vi "Digitalni osciloskop.vi"() -> ()   [LabVIEW 2014]
uses:
  <instrlib>/niScope/Controls/niScope scalar measurement.ctl
  <instrlib>/niScope/Acquire/Fetch/niScope Fetch WDT.vi
panel:
  out "error out":errorcluster
  in  "error in":errorcluster
  in  "Channel":string
  out "Amplitude":dbl
  out "Min voltage":dbl
  out "Max voltage":dbl
  out "VPP":dbl
  out "Frequency":dbl
  in  "Stop Button":bool
  in  "Save plot":bool
  in  "horizontal range":dbl(knob) scale=1000.0..100000.0
  in  "vertical range":dbl(knob) scale=0.0..10.0
  in  "Filter":u16(ring) items=["Both"=3, "Lowpass filter"=1, "None"=0, "Highpass filter"=2]
  in  "Highpass filter":dbl
  in  "Lowpass filter":dbl
  in  "Freeze/Stop":bool
  out "Waveform Graph":waveform(dbl)(graph)
  in  "resource name":refnum<k15>="DAQ::1" caption="Resource name"
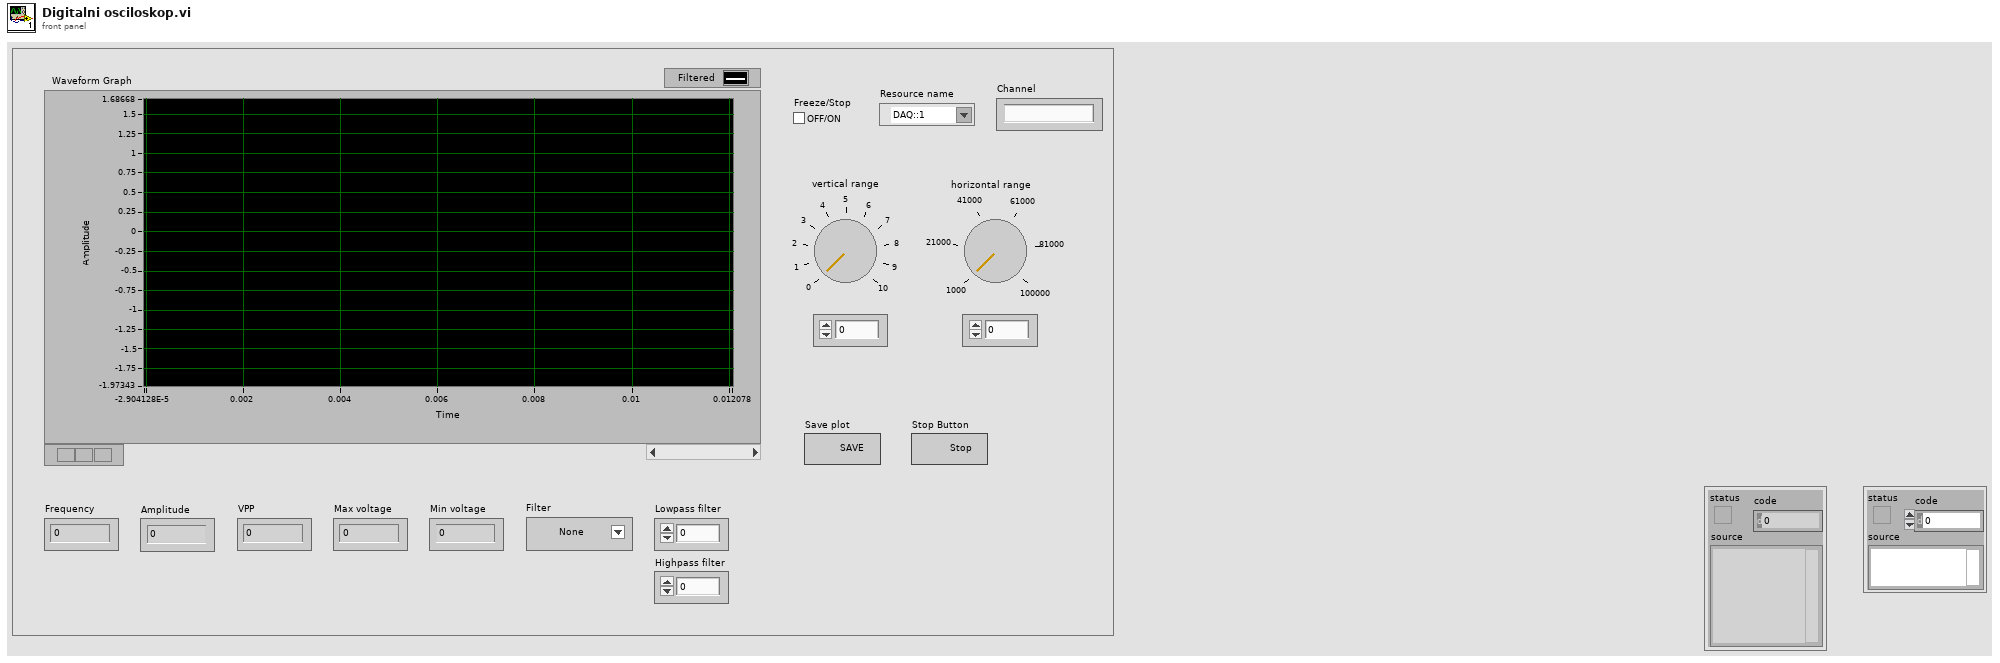
[diagram p1: front panel]
types:
  T1 = typedef "niScope scalar measurement.ctl" = i32
  T2 = typedef "imagedata.ctl" = cluster{"image type":i32, "image depth":i32, "image":u8[], "mask":u8[], "colors":u32[], "Rectangle":cluster{"left":i16, "top":i16, "right":i16, "bottom":i16}}
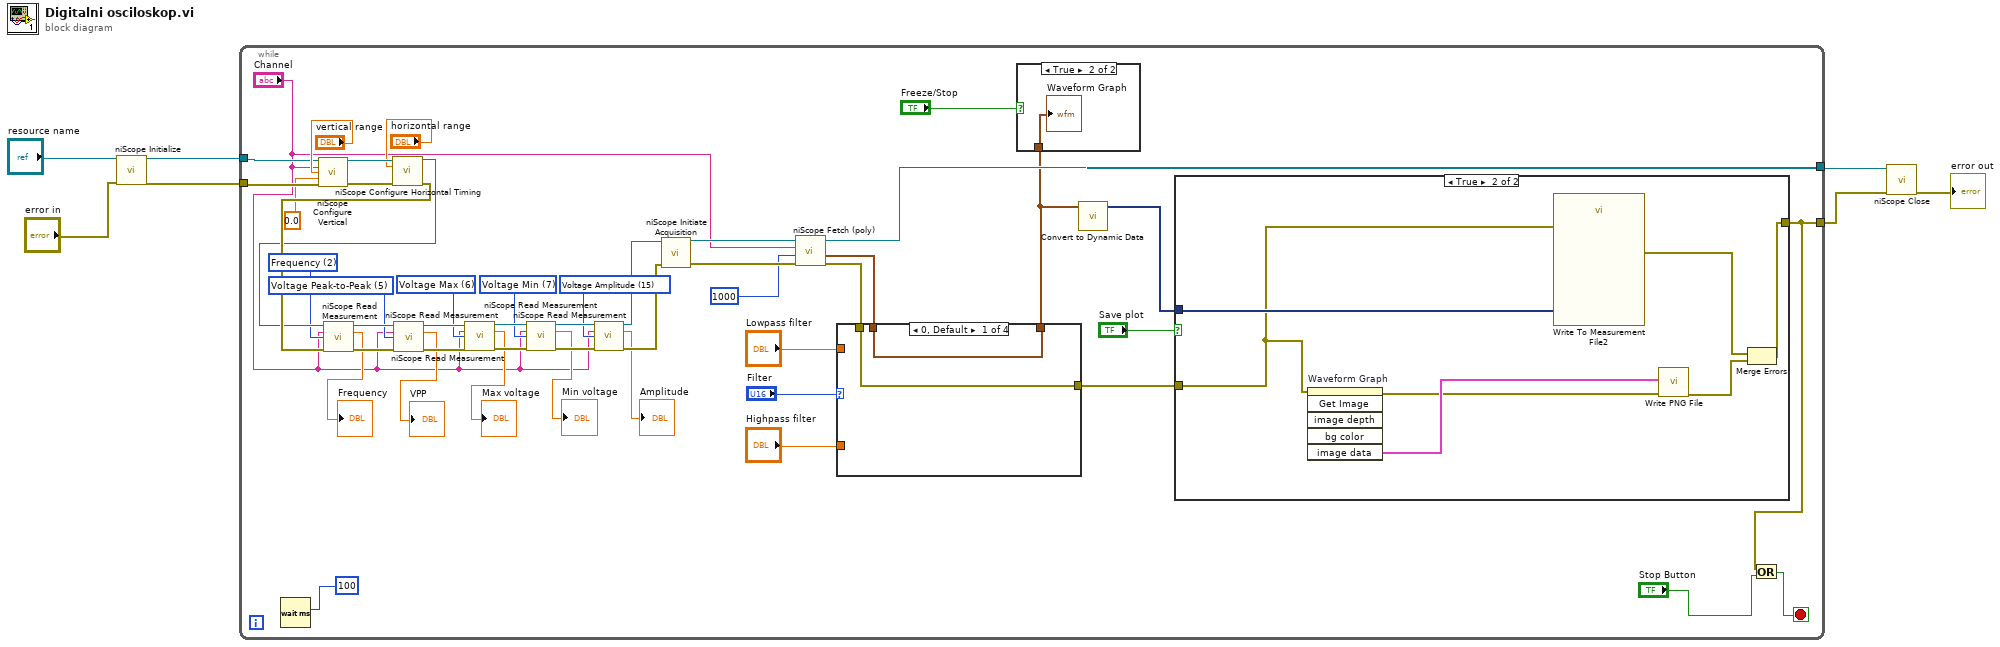
[diagram p0: block diagram]
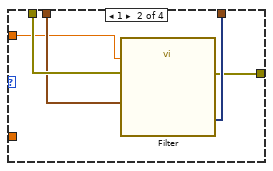
[diagram p4: hidden frame]
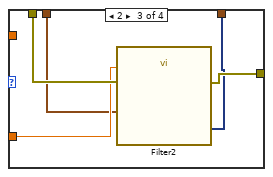
[diagram p5: hidden frame]
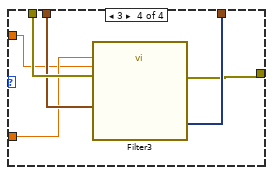
[diagram p6: hidden frame]
diagram:
  n1 = call <instrlib>:"niScope Initialize.vi"("resource name"="resource name", "error in"="error in") -> ("instrument handle"=w6:refnum<k15>, "error out"=w5:errorcluster)  [unwired: 12 in]
  n2 = while {
    tunnel: w6 -> [w43]
    tunnel: w5 -> [w44]
    tunnel: [w51] -> w4
    tunnel: [w10] -> w3
    stop <- w9 stop-if-true
    w25 = T1 15 items=["None"=4000, "Frequency"=2, "Average Frequency"=1016, "FFT Frequency"=1008, "Period"=3, "Average Period"=1015, "Rise Time"=0, "Fall Time"=1, "Rising Slew Rate"=1010, "Falling Slew Rate"=1011, "Overshoot"=18, "Preshoot"=19, "Voltage RMS"=4, "Voltage Cycle RMS"=16, "AC Estimate"=1012, "FFT Amplitude"=1009, "Voltage Average"=10, "Voltage Cycle Average"=17, "DC Estimate"=1013, "Voltage Max"=6, "Voltage Min"=7, "Voltage Peak-to-Peak"=5, "Voltage High"=8, "Voltage Low"=9, "Voltage Amplitude"=15, "Voltage Top"=1007, "Voltage Base"=1006, "Voltage Base-to-Top"=1017, "Negative Width"=11, "Positive Width"=12, "Negative Duty Cycle"=13, "Positive Duty Cycle"=14, "Integral"=1005, "Area"=1003, "Cycle Area"=1004, "Time Delay"=1014, "Phase Delay"=1018, "Low Ref Volts"=1000, "Mid Ref Volts"=1001, "High Ref Volts"=1002, "Volt. Hist. Mean"=2000, "Volt. Hist. Stdev"=2001, "Volt. Hist. Median"=2003, "Volt. Hist. Mode"=2010, "Volt. Hist. Max"=2005, "Volt. Hist. Min"=2006, "Volt. Hist. Peak-to-Peak"=2002, "Volt. Hist. Mean + Stdev"=2007, "Volt. Hist. Mean + 2 Stdev"=2008, "Volt. Hist. Mean + 3 Stdev"=2009, "Volt. Hist. Hits"=2004, "Volt. Hist. New Hits"=2011, "Time Hist. Mean"=3000, "Time Hist. Stdev"=3001, "Time Hist. Median"=3003, "Time Hist. Mode"=3010, "Time Hist. Max"=3005, "Time Hist. Min"=3006, "Time Hist. Peak-to-Peak"=3002, "Time Hist. Mean + Stdev"=3007, "Time Hist. Mean + 2 Stdev"=3008, "Time Hist. Mean + 3 Stdev"=3009, "Time Hist. Hits"=3004, "Time Hist. New Hits"=3011] ("scalar measurement")
    w26 = T1 7 items=["None"=4000, "Frequency"=2, "Average Frequency"=1016, "FFT Frequency"=1008, "Period"=3, "Average Period"=1015, "Rise Time"=0, "Fall Time"=1, "Rising Slew Rate"=1010, "Falling Slew Rate"=1011, "Overshoot"=18, "Preshoot"=19, "Voltage RMS"=4, "Voltage Cycle RMS"=16, "AC Estimate"=1012, "FFT Amplitude"=1009, "Voltage Average"=10, "Voltage Cycle Average"=17, "DC Estimate"=1013, "Voltage Max"=6, "Voltage Min"=7, "Voltage Peak-to-Peak"=5, "Voltage High"=8, "Voltage Low"=9, "Voltage Amplitude"=15, "Voltage Top"=1007, "Voltage Base"=1006, "Voltage Base-to-Top"=1017, "Negative Width"=11, "Positive Width"=12, "Negative Duty Cycle"=13, "Positive Duty Cycle"=14, "Integral"=1005, "Area"=1003, "Cycle Area"=1004, "Time Delay"=1014, "Phase Delay"=1018, "Low Ref Volts"=1000, "Mid Ref Volts"=1001, "High Ref Volts"=1002, "Volt. Hist. Mean"=2000, "Volt. Hist. Stdev"=2001, "Volt. Hist. Median"=2003, "Volt. Hist. Mode"=2010, "Volt. Hist. Max"=2005, "Volt. Hist. Min"=2006, "Volt. Hist. Peak-to-Peak"=2002, "Volt. Hist. Mean + Stdev"=2007, "Volt. Hist. Mean + 2 Stdev"=2008, "Volt. Hist. Mean + 3 Stdev"=2009, "Volt. Hist. Hits"=2004, "Volt. Hist. New Hits"=2011, "Time Hist. Mean"=3000, "Time Hist. Stdev"=3001, "Time Hist. Median"=3003, "Time Hist. Mode"=3010, "Time Hist. Max"=3005, "Time Hist. Min"=3006, "Time Hist. Peak-to-Peak"=3002, "Time Hist. Mean + Stdev"=3007, "Time Hist. Mean + 2 Stdev"=3008, "Time Hist. Mean + 3 Stdev"=3009, "Time Hist. Hits"=3004, "Time Hist. New Hits"=3011] ("scalar measurement")
    w27 = T1 6 items=["None"=4000, "Frequency"=2, "Average Frequency"=1016, "FFT Frequency"=1008, "Period"=3, "Average Period"=1015, "Rise Time"=0, "Fall Time"=1, "Rising Slew Rate"=1010, "Falling Slew Rate"=1011, "Overshoot"=18, "Preshoot"=19, "Voltage RMS"=4, "Voltage Cycle RMS"=16, "AC Estimate"=1012, "FFT Amplitude"=1009, "Voltage Average"=10, "Voltage Cycle Average"=17, "DC Estimate"=1013, "Voltage Max"=6, "Voltage Min"=7, "Voltage Peak-to-Peak"=5, "Voltage High"=8, "Voltage Low"=9, "Voltage Amplitude"=15, "Voltage Top"=1007, "Voltage Base"=1006, "Voltage Base-to-Top"=1017, "Negative Width"=11, "Positive Width"=12, "Negative Duty Cycle"=13, "Positive Duty Cycle"=14, "Integral"=1005, "Area"=1003, "Cycle Area"=1004, "Time Delay"=1014, "Phase Delay"=1018, "Low Ref Volts"=1000, "Mid Ref Volts"=1001, "High Ref Volts"=1002, "Volt. Hist. Mean"=2000, "Volt. Hist. Stdev"=2001, "Volt. Hist. Median"=2003, "Volt. Hist. Mode"=2010, "Volt. Hist. Max"=2005, "Volt. Hist. Min"=2006, "Volt. Hist. Peak-to-Peak"=2002, "Volt. Hist. Mean + Stdev"=2007, "Volt. Hist. Mean + 2 Stdev"=2008, "Volt. Hist. Mean + 3 Stdev"=2009, "Volt. Hist. Hits"=2004, "Volt. Hist. New Hits"=2011, "Time Hist. Mean"=3000, "Time Hist. Stdev"=3001, "Time Hist. Median"=3003, "Time Hist. Mode"=3010, "Time Hist. Max"=3005, "Time Hist. Min"=3006, "Time Hist. Peak-to-Peak"=3002, "Time Hist. Mean + Stdev"=3007, "Time Hist. Mean + 2 Stdev"=3008, "Time Hist. Mean + 3 Stdev"=3009, "Time Hist. Hits"=3004, "Time Hist. New Hits"=3011] ("scalar measurement")
    w28 = T1 5 items=["None"=4000, "Frequency"=2, "Average Frequency"=1016, "FFT Frequency"=1008, "Period"=3, "Average Period"=1015, "Rise Time"=0, "Fall Time"=1, "Rising Slew Rate"=1010, "Falling Slew Rate"=1011, "Overshoot"=18, "Preshoot"=19, "Voltage RMS"=4, "Voltage Cycle RMS"=16, "AC Estimate"=1012, "FFT Amplitude"=1009, "Voltage Average"=10, "Voltage Cycle Average"=17, "DC Estimate"=1013, "Voltage Max"=6, "Voltage Min"=7, "Voltage Peak-to-Peak"=5, "Voltage High"=8, "Voltage Low"=9, "Voltage Amplitude"=15, "Voltage Top"=1007, "Voltage Base"=1006, "Voltage Base-to-Top"=1017, "Negative Width"=11, "Positive Width"=12, "Negative Duty Cycle"=13, "Positive Duty Cycle"=14, "Integral"=1005, "Area"=1003, "Cycle Area"=1004, "Time Delay"=1014, "Phase Delay"=1018, "Low Ref Volts"=1000, "Mid Ref Volts"=1001, "High Ref Volts"=1002, "Volt. Hist. Mean"=2000, "Volt. Hist. Stdev"=2001, "Volt. Hist. Median"=2003, "Volt. Hist. Mode"=2010, "Volt. Hist. Max"=2005, "Volt. Hist. Min"=2006, "Volt. Hist. Peak-to-Peak"=2002, "Volt. Hist. Mean + Stdev"=2007, "Volt. Hist. Mean + 2 Stdev"=2008, "Volt. Hist. Mean + 3 Stdev"=2009, "Volt. Hist. Hits"=2004, "Volt. Hist. New Hits"=2011, "Time Hist. Mean"=3000, "Time Hist. Stdev"=3001, "Time Hist. Median"=3003, "Time Hist. Mode"=3010, "Time Hist. Max"=3005, "Time Hist. Min"=3006, "Time Hist. Peak-to-Peak"=3002, "Time Hist. Mean + Stdev"=3007, "Time Hist. Mean + 2 Stdev"=3008, "Time Hist. Mean + 3 Stdev"=3009, "Time Hist. Hits"=3004, "Time Hist. New Hits"=3011] ("scalar measurement")
    w39 = T1 2 items=["None"=4000, "Frequency"=2, "Average Frequency"=1016, "FFT Frequency"=1008, "Period"=3, "Average Period"=1015, "Rise Time"=0, "Fall Time"=1, "Rising Slew Rate"=1010, "Falling Slew Rate"=1011, "Overshoot"=18, "Preshoot"=19, "Voltage RMS"=4, "Voltage Cycle RMS"=16, "AC Estimate"=1012, "FFT Amplitude"=1009, "Voltage Average"=10, "Voltage Cycle Average"=17, "DC Estimate"=1013, "Voltage Max"=6, "Voltage Min"=7, "Voltage Peak-to-Peak"=5, "Voltage High"=8, "Voltage Low"=9, "Voltage Amplitude"=15, "Voltage Top"=1007, "Voltage Base"=1006, "Voltage Base-to-Top"=1017, "Negative Width"=11, "Positive Width"=12, "Negative Duty Cycle"=13, "Positive Duty Cycle"=14, "Integral"=1005, "Area"=1003, "Cycle Area"=1004, "Time Delay"=1014, "Phase Delay"=1018, "Low Ref Volts"=1000, "Mid Ref Volts"=1001, "High Ref Volts"=1002, "Volt. Hist. Mean"=2000, "Volt. Hist. Stdev"=2001, "Volt. Hist. Median"=2003, "Volt. Hist. Mode"=2010, "Volt. Hist. Max"=2005, "Volt. Hist. Min"=2006, "Volt. Hist. Peak-to-Peak"=2002, "Volt. Hist. Mean + Stdev"=2007, "Volt. Hist. Mean + 2 Stdev"=2008, "Volt. Hist. Mean + 3 Stdev"=2009, "Volt. Hist. Hits"=2004, "Volt. Hist. New Hits"=2011, "Time Hist. Mean"=3000, "Time Hist. Stdev"=3001, "Time Hist. Median"=3003, "Time Hist. Mode"=3010, "Time Hist. Max"=3005, "Time Hist. Min"=3006, "Time Hist. Peak-to-Peak"=3002, "Time Hist. Mean + Stdev"=3007, "Time Hist. Mean + 2 Stdev"=3008, "Time Hist. Mean + 3 Stdev"=3009, "Time Hist. Hits"=3004, "Time Hist. New Hits"=3011] ("scalar measurement")
    n3 = Wait (ms)(milliseconds to wait=u32 100) -> ()  [unwired: 1 out]
    n4 = call <instrlib>:"niScope Configure Vertical.vi"("instrument handle"=w43, "channels"="Channel", "vertical range"="vertical range", "vertical offset"=0.0, "error in"=w44) -> ("instrument handle out"=w46:refnum<k15>, "error out"=w42:errorcluster)  [unwired: 9 in]
    n5 = call <instrlib>:"niScope Configure Horizontal Timing.vi"("instrument handle"=w46, "min sample rate"="horizontal range", "error in"=w42) -> ("instrument handle out"=w40:refnum<k15>, "error out"=w41:errorcluster)  [unwired: 11 in]
    n6 = call <instrlib>:"niScope Read Measurement.vi"("instrument handle"=w40, "channels"="Channel", "scalar measurement"=w39, "error in"=w41) -> ("instrument handle out"=w34:refnum<k15>, "result"=→"Frequency":dbl, "error out"=w38:errorcluster)  [unwired: 9 in]
    n7 = call <instrlib>:"niScope Read Measurement.vi"("instrument handle"=w34, "channels"="Channel", "scalar measurement"=w28, "error in"=w38) -> ("instrument handle out"=w33:refnum<k15>, "result"=→"VPP":dbl, "error out"=w37:errorcluster)  [unwired: 9 in]
    n8 = call <instrlib>:"niScope Read Measurement.vi"("instrument handle"=w33, "channels"="Channel", "scalar measurement"=w27, "error in"=w37) -> ("instrument handle out"=w32:refnum<k15>, "result"=→"Max voltage":dbl, "error out"=w36:errorcluster)  [unwired: 9 in]
    n9 = call <instrlib>:"niScope Read Measurement.vi"("instrument handle"=w32, "channels"="Channel", "scalar measurement"=w26, "error in"=w36) -> ("instrument handle out"=w31:refnum<k15>, "result"=→"Min voltage":dbl, "error out"=w35:errorcluster)  [unwired: 9 in]
    n10 = call <instrlib>:"niScope Read Measurement.vi"("instrument handle"=w31, "channels"="Channel", "scalar measurement"=w25, "error in"=w35) -> ("instrument handle out"=w30:refnum<k15>, "result"=→"Amplitude":dbl, "error out"=w29:errorcluster)  [unwired: 9 in]
    n11 = call <instrlib>:"niScope Initiate Acquisition.vi"("instrument handle"=w30, "error in"=w29) -> ("instrument handle out"=w54:refnum<k15>, "error out"=w53:errorcluster)  [unwired: 12 in]
    n12 = call-poly <instrlib>:"niScope Fetch (poly).vi"("error in"=w53, "numSamples"=1000, "channels"="Channel", "instrument handle"=w54) -> ("error out"=w50:errorcluster, "wfm"=w14:waveform(dbl), "instrument handle out"=w51:refnum<k15>)  [unwired: 4 in, 1 out]
    n13 = case shown="0, Default" "Filter" {
      tunnel: w50 -> [w65 w71 w76 w82]
      tunnel: w14 -> [w66 w70 w74 w81]
      tunnel: [w66 w69 w72 w78] -> w13
      tunnel: [w65 w68 w73 w77] -> w12
      tunnel: "Lowpass filter" -> [_ w67 _ w79]
      tunnel: "Highpass filter" -> [_ _ w75 w80]
      frame 0, Default {
      }
      frame 1 {
        n14 = call "Filter"("error in (no error)"=w71, "Lower Cut-Off"=w67, "Signal"=w70) -> ("error out"=w68:errorcluster, "Filtered Signal"=w69:dynamicdata)  [unwired: 7 in]
      }
      frame 2 {
        n15 = call "Filter2"("error in (no error)"=w76, "Lower Cut-Off"=w75, "Signal"=w74) -> ("error out"=w73:errorcluster, "Filtered Signal"=w72:dynamicdata)  [unwired: 7 in]
      }
      frame 3 {
        n16 = call "Filter3"("error in (no error)"=w82, "Lower Cut-Off"=w79, "Upper Cut-Off"=w80, "Signal"=w81) -> ("error out"=w77:errorcluster, "Filtered Signal"=w78:dynamicdata)  [unwired: 6 in]
      }
    }
    n17 = case shown="True" "Freeze/Stop" {
      tunnel: w13 -> [_ w64]
      frame False {
      }
      frame True {
        "Waveform Graph" <- w64
      }
    }
    n18 = call "Convert to Dynamic Data"("Array"=w13) -> ("Dynamic Data Type"=w15:dynamicdata)  [unwired: 3 in]
    n19 = case shown="True" "Save plot" {
      tunnel: [w56 w57] -> w10
      tunnel: w15 -> [_ w63]
      tunnel: w12 -> [w56 w61]
      frame False {
      }
      frame True {
        n20 = invoke on="Waveform Graph" class="WFGraph (strict)" method="Get Image"(error in=w61) -> (error out=w60:errorcluster, "image data"=w62:T2)  [unwired: 5 in, 4 out]
        n21 = call "Write To Measurement File2"("Signals"=w63, "error in (no error)"=w61) -> ("error out"=w58:errorcluster)  [unwired: 15 in, 2 out]
        n22 = call <vilib>:"Write PNG File.vi"("error in (no error)"=w60, "image data"=w62) -> ("error out"=w59:errorcluster)  [unwired: 8 in, 1 out]
        n23 = Merge Errors(w58, w59) -> (w57:errorcluster)
      }
    }
    n24 = Or(x=w10, y="Stop Button") -> (x .or. y?=w9:bool)
  }
  n25 = call <instrlib>:"niScope Close.vi"("instrument handle"=w4, "error in"=w3) -> ("error out"=→"error out":errorcluster)  [unwired: 13 in]
